vi "CalculateXYZ.vi"(1 "CMF":dbl[][](array[numeric]), 2 "Reflectance":dbl[](array[numeric]), 3 "Illuminant":dbl[](array[numeric])) -> (0 "XYZ":dbl[](array[numeric]))   [LabVIEW 2013]
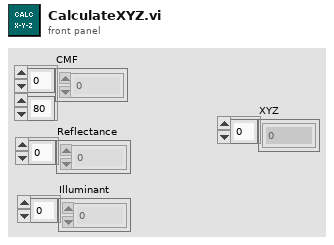
[diagram p1: front panel]
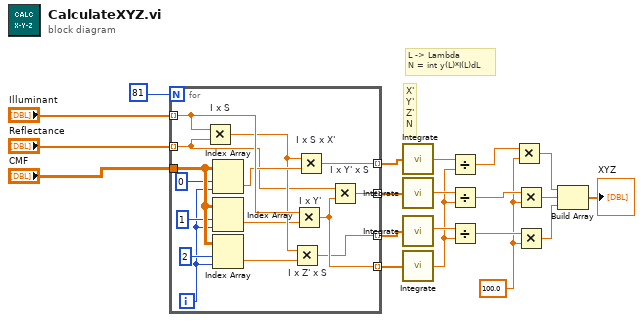
[diagram p0: block diagram]
diagram:
  w5 = 100.0 ("y")
  # "X'\nY'\nZ'\nN"
  # "L -> Lambda\nN = int y(L)*I(L)dL"
  n1 = for {
    N: 81 -> [_]
    tunnel: "CMF" -> [w35]
    tunnel: "Illuminant" -> [w34] mode=indexing
    tunnel: "Reflectance" -> [w30] mode=indexing
    tunnel: [w29] -> w9 mode=indexing
    tunnel: [w28] -> w11 mode=indexing
    tunnel: [w27] -> w12 mode=indexing
    tunnel: [w26] -> w10 mode=indexing
    i -> [w22]
    n2 = Multiply "I x S"(x=w34, y=w30) -> (x*y=w32:dbl)
    n3 = Index Array(array=w35, index (row)=0 ("disabled index (col)"), index (col)=w22) -> (element=w33:dbl)
    n4 = Index Array(array=w35, index (row)=1 ("disabled index (col)"), index (col)=w22) -> (element=w31:dbl)
    n5 = Index Array(array=w35, index (row)=2 ("disabled index (col)"), index (col)=w22) -> (element=w21:dbl)
    n6 = Multiply "I x Z' x S"(x=w32, y=w21) -> (x*y=w26:dbl)
    n7 = Multiply "I x Y'"(x=w34, y=w31) -> (x*y=w29:dbl)
    n8 = Multiply "I x S x X'"(x=w32, y=w33) -> (x*y=w27:dbl)
    n9 = Multiply "I x Y' x S"(x=w30, y=w29) -> (x*y=w28:dbl)
  }
  n10 = call "Integrate.vi"("Array"=w12) -> ("Integral result"=w19:dbl)
  n11 = call "Integrate.vi"("Array"=w11) -> ("Integral result"=w18:dbl)
  n12 = call "Integrate.vi"("Array"=w10) -> ("Integral result"=w17:dbl)
  n13 = call "Integrate.vi"("Array"=w9) -> ("Integral result"=w16:dbl)
  n14 = Divide(x=w19, y=w16) -> (x/y=w8:dbl)
  n15 = Divide(x=w18, y=w16) -> (x/y=w7:dbl)
  n16 = Divide(x=w17, y=w16) -> (x/y=w6:dbl)
  n17 = Multiply(x=w8, y=w5) -> (x*y=w4:dbl)
  n18 = Multiply(x=w7, y=w5) -> (x*y=w3:dbl)
  n19 = Multiply(x=w6, y=w5) -> (x*y=w2:dbl)
  n20 = Build Array(w4, w3, w2) -> (→"XYZ":dbl[])
